vi "Read Configuration Parameters.vi"(8 "error in (no error)":errorcluster, 10 "refnum":T1, 11 "DAQ Configuration in":refnum<class "DAQ Configuration.lvclass">) -> (0 "error out":errorcluster, 2 "refnum out":T1, 3 "DAQ Configuration out":refnum<class "DAQ Configuration.lvclass">)   [LabVIEW 2026, in "Hardware.lvlib" / "DAQ Configuration.lvclass"]
uses:
  DAQ Configuration.lvclass
  <vilib>/Utility/config.llb/Config Data RefNum.ctl
  DAQ Configuration.lvclass/DAQ Configuration.ctl
  framework/Hardware/HW with output config.lvclass
  <vilib>/Utility/config.llb/NI_LVConfig.lvlib
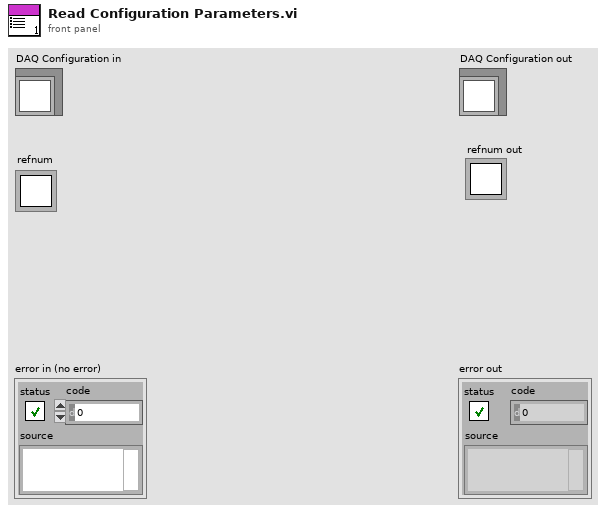
[diagram p1: front panel]
types:
  T1 = typedef "NI_LVConfig.lvlib/Config Data RefNum.ctl" = refnum<k1>
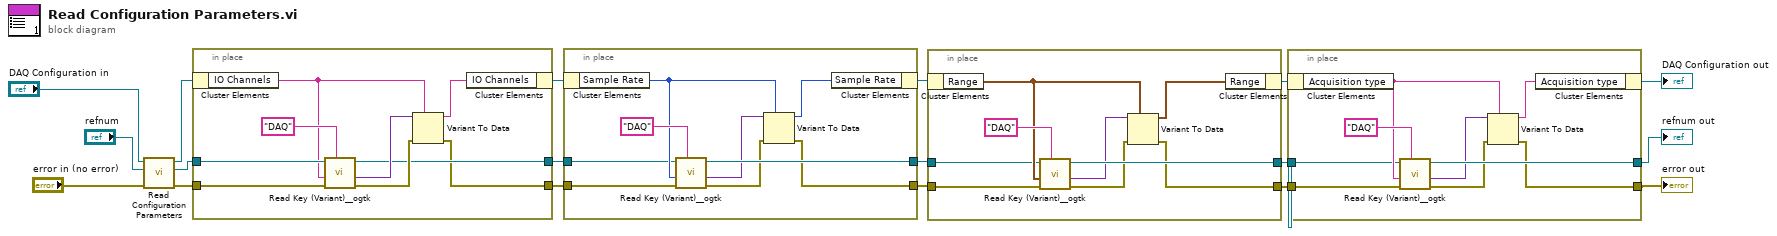
[diagram p0: block diagram]
diagram:
  n1 = call-parent "Read Configuration Parameters.vi"("error in (no error)"="error in (no error)", "refnum"="refnum", "HW with output config in"="DAQ Configuration in") -> ("error out"=w10:errorcluster, "refnum out"=w11:T1, "HW with output config out"=w12:refnum<class "DAQ Configuration.lvclass">)  [unwired: 6 in]
  n2 = in-place "In Place Element Structure" {
    in-place-border: w11 -> [w25]
    in-place-border: w10 -> [w19]
    in-place-border: [w23] -> w14
    in-place-border: [w22] -> w13
    n3 = in-place-cluster #1(w12) -> ("IO Channels"=w21:string)
    n4 = call <userlib>:"Read Key (Variant)__ogtk.vi"("section"="DAQ", "error in (no error)"=w19, "type"=w21, "refnum"=w25) -> ("error out"=w26:errorcluster, "key-value"=w27:variant, "refnum out"=w23:T1)  [unwired: 4 in, 1 out]
    n5 = Variant To Data(error in=w26, type=w21, Variant=w27) -> (data=w20:string, error out=w22:errorcluster)
    n6 = in-place-cluster #1("IO Channels"=w20) -> (w15:refnum<class "DAQ Configuration.lvclass">)
  }
  n7 = in-place "In Place Element Structure" {
    in-place-border: [w30] -> w9
    in-place-border: [w35] -> w8
    in-place-border: w14 -> [w29]
    in-place-border: w13 -> [w28]
    n8 = in-place-cluster #2(w15) -> ("Sample Rate"=w34:i32)
    n9 = call <userlib>:"Read Key (Variant)__ogtk.vi"("section"="DAQ", "error in (no error)"=w28, "type"=w34, "refnum"=w29) -> ("error out"=w31:errorcluster, "key-value"=w33:variant, "refnum out"=w35:T1)  [unwired: 4 in, 1 out]
    n10 = Variant To Data(error in=w31, type=w34, Variant=w33) -> (data=w32:i32, error out=w30:errorcluster)
    n11 = in-place-cluster #2("Sample Rate"=w32) -> (w7:refnum<class "DAQ Configuration.lvclass">)
  }
  n12 = in-place "In Place Element Structure" {
    in-place-border: [w39] -> w5
    in-place-border: [w44] -> w6
    in-place-border: w8 -> [w38]
    in-place-border: w9 -> [w37]
    n13 = in-place-cluster #3(w7) -> ("Range"=w43:cluster{"Ranve (min)":dbl, "Range Max":dbl})
    n14 = call <userlib>:"Read Key (Variant)__ogtk.vi"("section"="DAQ", "error in (no error)"=w37, "type"=w43, "refnum"=w38) -> ("error out"=w40:errorcluster, "key-value"=w42:variant, "refnum out"=w44:T1)  [unwired: 4 in, 1 out]
    n15 = Variant To Data(error in=w40, type=w43, Variant=w42) -> (data=w41:cluster{"Ranve (min)":dbl, "Range Max":dbl}, error out=w39:errorcluster)
    n16 = in-place-cluster #3("Range"=w41) -> (w4:refnum<class "DAQ Configuration.lvclass">)
  }
  n17 = in-place "In Place Element Structure" {
    in-place-border: [w48] -> w1
    in-place-border: [w53] -> w2
    in-place-border: w6 -> [w47]
    in-place-border: w5 -> [w46]
    n18 = in-place-cluster #4(w4) -> ("Acquisition type"=w52:string)
    n19 = call <userlib>:"Read Key (Variant)__ogtk.vi"("section"="DAQ", "error in (no error)"=w46, "type"=w52, "refnum"=w47) -> ("error out"=w49:errorcluster, "key-value"=w51:variant, "refnum out"=w53:T1)  [unwired: 4 in, 1 out]
    n20 = Variant To Data(error in=w49, type=w52, Variant=w51) -> (data=w50:string, error out=w48:errorcluster)
    n21 = in-place-cluster #4("Acquisition type"=w50) -> (→"DAQ Configuration out":refnum<class "DAQ Configuration.lvclass">)
  }
  "error out" <- w1
  "refnum out" <- w2
